vi "Outputs.vi"(1 "error in (no error)":errorcluster, 2 "Value":i16) -> (0 "error out":errorcluster)   [LabVIEW 2013]
doc: "Use this template to build a VI to use as a subVI."
uses:
  704IO.dll
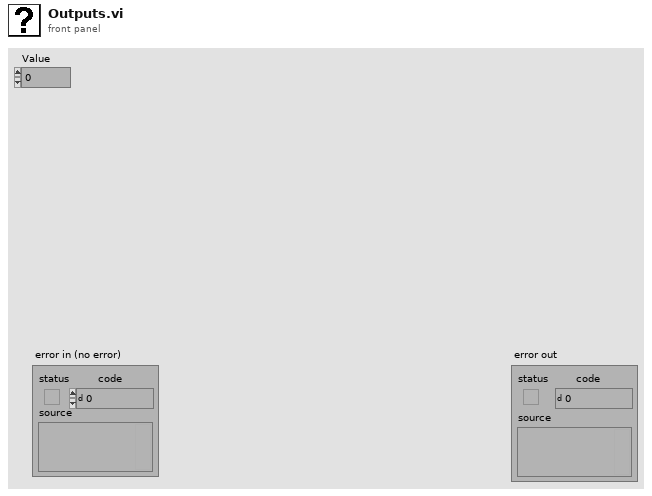
[diagram p1: front panel]
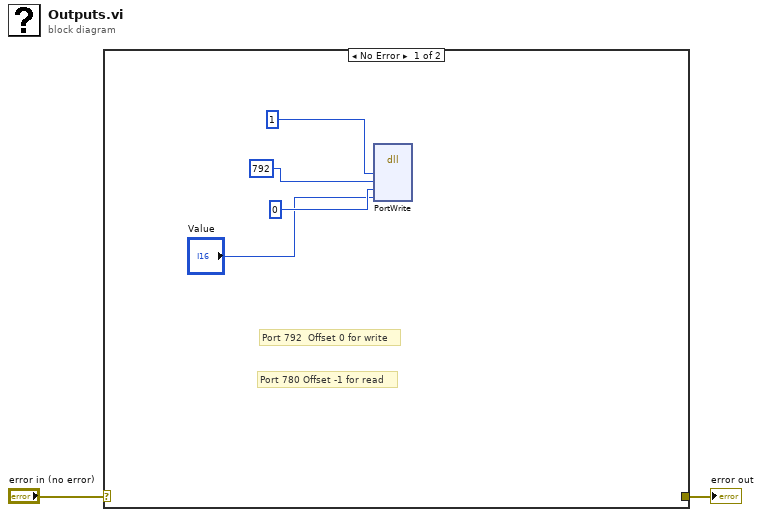
[diagram p0: block diagram]
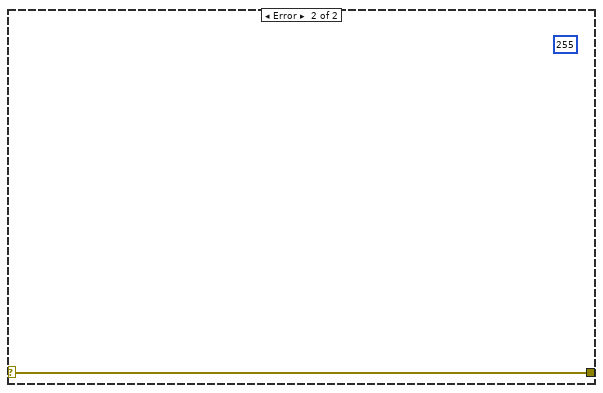
[diagram p2: hidden frame]
diagram:
  n1 = case shown="No Error" "error in (no error)" {
    selector: "error in (no error)" -> [_ w7]
    tunnel: [_ w7] -> w1
    frame No Error {
      # "Port 780 Offset -1 for read"
      # "Port 792  Offset 0 for write"
      n2 = dll-call lib="C:/Users/Radu Darie/Documents/GitHub/ParkinsonsCorridor/704IO.dll" fn="PortWrite"("Rack"=i16 1 ("Port"), "Port"=i16 792 ("Rack"), "Offset"=i16 0, "Value"="Value") -> ()  [unwired: 8 in, 2 out]
    }
    frame Error {
      (unwired) i16 255 ("return type")
    }
  }
  "error out" <- w1
